vi "PDCAVISave.vi"(0 "DeviceNo":u32, 1 "FileName":string, 2 "Slide Refnum":refnum<vi>, 5 "ChildNo":u32, 9 "Rate":i32=30, 11 "error in (no error)":errorcluster, 12 "ShowCompreddDlg":u32, 13 "File_Frame":cluster{"StartFrame":i32, "EndFrame":i32}) -> (15 "error out":errorcluster)   [LabVIEW 2015]
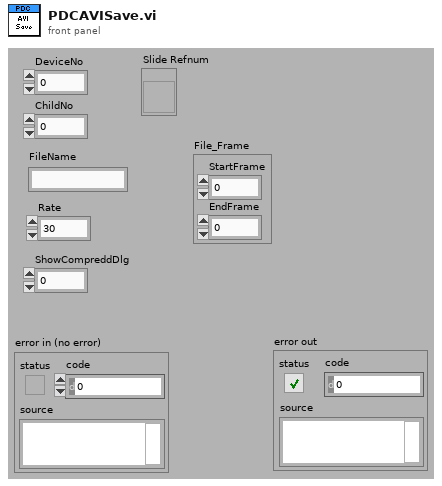
[diagram p1: front panel]
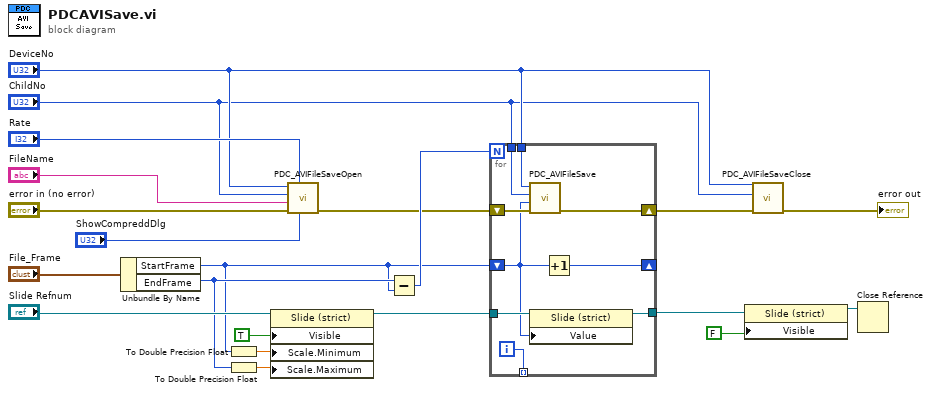
[diagram p0: block diagram]
diagram:
  n1 = Unbundle By Name("File_Frame") -> ("StartFrame"=w1:i32, "EndFrame"=w2:i32)
  n2 = To Double Precision Float(number=w1) -> (double precision float=w15:dbl)
  n3 = To Double Precision Float(number=w2) -> (double precision float=w16:dbl)
  n4 = property class="Slide (strict)"(reference="Slide Refnum", "Visible"=TRUE ("表示"), "Scale.Minimum"=w15, "Scale.Maximum"=w16) -> (reference out=w3:refnum<vi>)  [unwired: 1 in, 1 out]
  n5 = call "PDC_AVIFileSaveOpen.vi"("ShowCompressDlg"="ShowCompreddDlg", "Rate"="Rate", "error in (no error)"="error in (no error)", "FileName"="FileName", "ChildNo"="ChildNo", "DeviceNo"="DeviceNo") -> ("error out"=w5:errorcluster)  [unwired: 5 out]
  n6 = Subtract(x=w2, y=w1) -> (x-y=w7:i32)
  n7 = for {
    N: w7 -> [_]
    tunnel: "DeviceNo" -> [w28]
    tunnel: "ChildNo" -> [w27]
    shift-right: [w26] -> _
    shift-left: w1 -> [w24]
    tunnel: w3 -> [w25]
    tunnel: [w23] -> w18
    tunnel: [w22] -> _ mode=indexing
    shift-right: [w29] -> w6
    shift-left: w5 -> [w30]
    i -> [w22]
    n8 = call "PDC_AVIFileSave.vi"("error in (no error)"=w30, "FrameNo"=w24, "ChildNo"=w27, "DeviceNo"=w28) -> ("error out"=w29:errorcluster)  [unwired: 7 out]
    n9 = property class="Slide (strict)"(reference=w25, "Value"=w24) -> (reference out=w23:refnum<vi>)  [unwired: 1 in, 1 out]
    n10 = Increment(x=w24) -> (x+1=w26:i32)
  }
  n11 = property class="Slide (strict)"(reference=w18, "Visible"=FALSE ("表示")) -> (reference out=w20:refnum<vi>)  [unwired: 1 in, 1 out]
  n12 = call "PDC_AVIFileSaveClose.vi"("error in (no error)"=w6, "ChildNo"="ChildNo", "DeviceNo"="DeviceNo") -> ("error out"=→"error out":errorcluster)  [unwired: 8 out]
  n13 = Close Reference(reference=w20) -> ()  [unwired: 1 in, 1 out]
